vi "XML Get Paths.vi"(0 "XML File Path In":path, 11 "Error In":errorcluster) -> (4 "XML File Path Out":path, 6 "Correction Period":u32, 8 "Response Matrix Path":path, 10 "Reference Orbit Path":path, 15 "Error Out":errorcluster)   [LabVIEW 2011, in "XML VIs.lvlib"]
uses:
  XML VIs.lvlib
  Third Party/GXML/_subVIis/GXML SearchParser/gxml_SearchParser.vi
  Third Party/GXML/GXML.lvlib
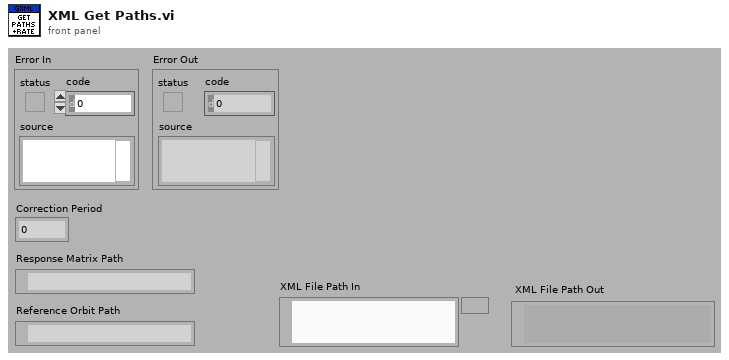
[diagram p1: front panel]
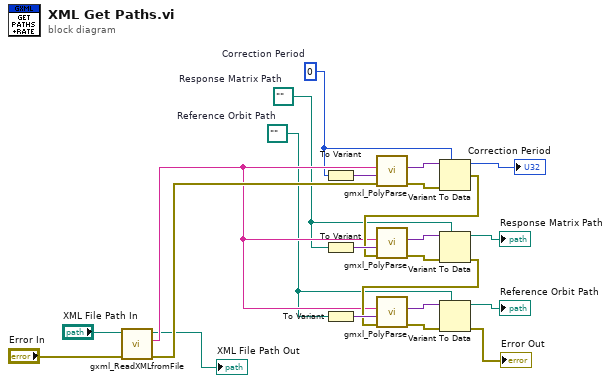
[diagram p0: block diagram]
diagram:
  w3 = u32 0  # Correction Period
  w4 = path ""  # Reference Orbit Path
  w5 = path ""  # Response Matrix Path
  n1 = call "gxml_ReadXMLfromFile.vi"("error in"="Error In", "XML File Path"="XML File Path In") -> ("error out"=w13:errorcluster, "XML String Out"=w10:string, "XML File Path Out"=→"XML File Path Out":path)  [unwired: 7 in]
  n2 = To Variant(anything=w3) -> (Variant=w21:variant)
  n3 = To Variant(anything=w5) -> (Variant=w19:variant)
  n4 = To Variant(anything=w4) -> (Variant=w14:variant)
  n5 = call-poly "gmxl_PolyParse.vi"("error in"=w13, "TypeDesc"=w21, "XML String In"=w10) -> ("error out"=w23:errorcluster, "Parsed Data"=w22:variant)  [unwired: 7 in]
  n6 = Variant To Data(error in=w23, type=w3, Variant=w22) -> (data=→"Correction Period":u32, error out=w12:errorcluster)
  n7 = call-poly "gmxl_PolyParse.vi"("error in"=w12, "TypeDesc"=w19, "XML String In"=w10) -> ("error out"=w17:errorcluster, "Parsed Data"=w18:variant)  [unwired: 7 in]
  n8 = Variant To Data(error in=w17, type=w5, Variant=w18) -> (data=→"Response Matrix Path":path, error out=w11:errorcluster)
  n9 = call-poly "gmxl_PolyParse.vi"("error in"=w11, "TypeDesc"=w14, "XML String In"=w10) -> ("error out"=w16:errorcluster, "Parsed Data"=w15:variant)  [unwired: 7 in]
  n10 = Variant To Data(error in=w16, type=w4, Variant=w15) -> (data=→"Reference Orbit Path":path, error out=→"Error Out":errorcluster)
